vi "Read Strings.vi"(9 "NamedNumeric in":refnum<class "NamedNumeric.lvclass">) -> (3 "NamedNumeric out":refnum<class "NamedNumeric.lvclass">, 4 "Strings":string[](array[string]))   [LabVIEW 2014, in "NamedNumeric.lvclass"]
uses:
  NamedNumeric.lvclass
  NamedNumeric.lvclass/NamedNumeric.ctl
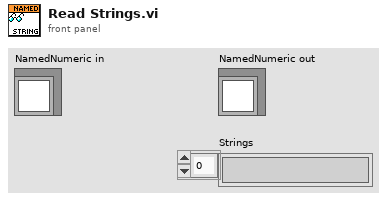
[diagram p1: front panel]
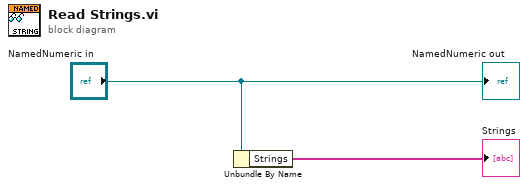
[diagram p0: block diagram]
diagram:
  n1 = Unbundle By Name("NamedNumeric in") -> ("Strings"=→"Strings":string[])
  "NamedNumeric out" <- "NamedNumeric in"
